vi "generatesquarewaveform.vi"() -> (0 "Waveform":waveform(dbl))   [LabVIEW 2015]
uses:
  <vilib>/measure/NI_MABase.lvlib
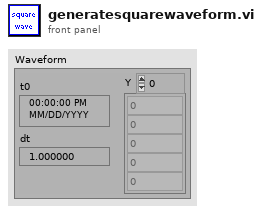
[diagram p1: front panel]
types:
  T1 = cluster{"AO parameters":cluster{"Build analog waveform tabs":dbl, "Repeats":dbl, "Cycles":dbl, "Start amplitude (V)":dbl, "Baseline (V)":dbl, "Step size (V)":dbl, "DC (%)":dbl, "Sampling frequency (Hz)":dbl, "Period (ms)":dbl, "Offset (V)":dbl, "Amplitude (V)":dbl, "Frequency":dbl, "Tri Repeats":dbl, "Cycle length (s)":dbl, "Pulses":dbl, "Matlab wave number":dbl}[], "DO parameters":cluster{"Digital DC (%)":dbl, "Digital phase":dbl, "Digital Freq (Hz)":dbl, "Sampling frequency (Hz)":dbl}[]}
  T2 = cluster{"VtoP":sgl[], "CWlasers":sgl[], "shutter":sgl[], "488":sgl[], "532":sgl[], "640":sgl[], "LT marker":sgl[]}
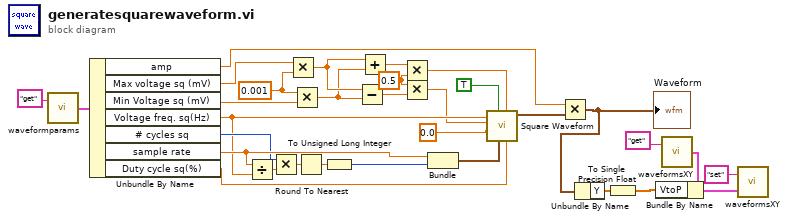
[diagram p0: block diagram]
diagram:
  w17 = 0.001
  w12 = 0.5 ("y")
  n1 = call "waveformparams.vi"("command"="get") -> ("Params out"=w28:T1)  [unwired: 1 in]
  n2 = Unbundle By Name(w28) -> ("amp"=w8:dbl, "Max voltage sq (mV)"=w16:dbl, "Min Voltage sq (mV)"=w18:dbl, "Voltage freq. sq(Hz)"=w24:dbl, "# cycles sq"=w25:u32, "sample rate"=w27:dbl, "Duty cycle sq(%)"=w21:dbl)
  n3 = Divide(x=w27, y=w24) -> (x/y=w26:dbl)
  n4 = Multiply(x=w25, y=w26) -> (x*y=w32:dbl)
  n5 = Multiply(x=w16, y=w17) -> (x*y=w15:dbl)
  n6 = Multiply(x=w17, y=w18) -> (x*y=w14:dbl)
  n7 = Round To Nearest(number=w32) -> (nearest integer value=w31:dbl)
  n8 = To Unsigned Long Integer(number=w31) -> (unsigned 32bit integer=w30:u32)
  n9 = Subtract(x=w15, y=w14) -> (x-y=w11:dbl)
  n10 = Add(x=w15, y=w14) -> (x+y=w13:dbl)
  n11 = Multiply(x=w13, y=w12) -> (x*y=w10:dbl)
  n12 = Multiply(x=w12, y=w11) -> (x*y=w9:dbl)
  n13 = Bundle("sample rate"=w27, w30) -> (w22:cluster{"sample rate":dbl, u32})  [unwired: 1 out]
  n14 = call <vilib>:"Square Waveform.vi"("duty cycle (%)"=w21, "offset"=w10, "sampling info"=w22, "reset signal"=TRUE, "phase"=0.0, "amplitude"=w9, "frequency"=w24) -> ("signal out"=w19:waveform(dbl))  [unwired: 3 in, 1 out]
  n15 = Multiply(x=w8, y=w19) -> (x*y=w4:waveform(dbl))
  "Waveform" <- w4
  n16 = Unbundle By Name(w4) -> ("Y"=w3:dbl[])
  n17 = To Single Precision Float(number=w3) -> (single precision float=w1:sgl[])
  n18 = call "waveformsXY.vi"("command"="get") -> ("waveforms out"=w5:T2)  [unwired: 1 in]
  n19 = Bundle By Name(cluster=w5, "VtoP"=w1) -> (w2:T2)
  n20 = call "waveformsXY.vi"("waveforms in"=w2, "command"="set") -> ()  [unwired: 1 out]
